vi "Is VI Server Required.vi"(8 "error in (no error)":errorcluster, 11 "Window Action in":refnum<class "Window Action.lvclass">) -> (0 "error out":errorcluster, 2 "VI Server Required?":bool, 3 "Window Action out":refnum<class "Window Action.lvclass">)   [LabVIEW 2020, in "MacroAssert.lvlib" / "Window Action.lvclass"]
doc: "Outputs whether VI Server is required to perform the given step."
uses:
  Window Action.lvclass
  Window Action.lvclass/Window Action.ctl
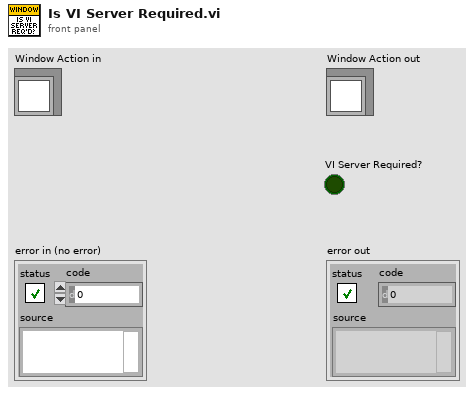
[diagram p1: front panel]
types:
  T1 = typedef "MacroAssert.lvlib/Window Action.lvclass/Window Action Type.ctl" = enum16{"Maximize Window", "Restore Window", "Minimize Window", "Close Window", "Bring Window to Front", "Send Window to Back"}
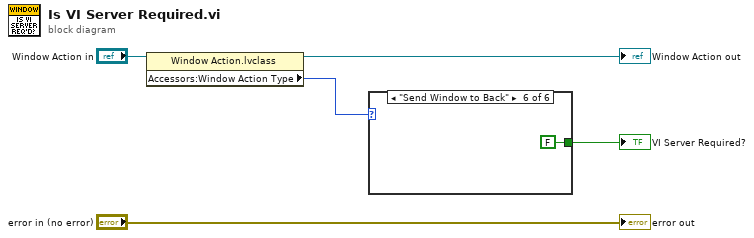
[diagram p0: block diagram]
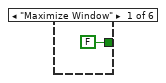
[diagram p2: hidden frame]
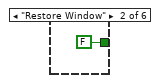
[diagram p3: hidden frame]
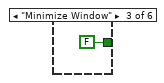
[diagram p4: hidden frame]
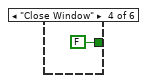
[diagram p5: hidden frame]
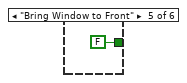
[diagram p6: hidden frame]
diagram:
  n1 = property class="Window Action.lvclass"(reference="Window Action in") -> (reference out=→"Window Action out":refnum<class "Window Action.lvclass">, "Accessors:Window Action Type"=w4:T1)  [unwired: 1 in, 1 out]
  n2 = case shown="\"Send Window to Back\"" w4 {
    tunnel: [FALSE FALSE FALSE FALSE FALSE FALSE] -> w2
    frame "Maximize Window" {
    }
    frame "Restore Window" {
    }
    frame "Minimize Window" {
    }
    frame "Close Window" {
    }
    frame "Bring Window to Front" {
    }
    frame "Send Window to Back" {
    }
  }
  "VI Server Required?" <- w2
  "error out" <- "error in (no error)"
